vi "DFD FXP MRate Modeling.vi"(4 "internal precision":T3, 5 "output integer word length":T1, 6 "output rounding mode":T2=enum."Truncation", 7 "input integer word length":i16=1, 8 "error in (no error)":errorcluster, 9 "output word length":i16=16, 10 "input word length":i16=16, 11 "multirate filter in":T4={"mMRate_Structure"=enum."IIR", "mMRate_Mode"=0, "mMRate_Factor"=-1, "mMRate_FIRParams"={"mMRate_FIR_H"=[], "mMRate_FIR_IsNyquist?"=FALSE, "mMRate_FIR_IsSymmetric?"=FALSE}, "mMRate_CICParams"={"mMRate_CIC_#Stage"=0, "mMRate_CIC_Lag"=0, "mMRate_CIC_Type"=enum."Lowpass"}, "mMRate_Order"=0, "mMRate_Version"="2.0", "mMRate_Comments"="", "mMRate_RationalFactor"={"mMRate_L"=-1, "mMRate_M"=-1}, "mMRate_Fs"=1.0, "mMRate_Quantized?"=FALSE, "mMRate_QFilterGain"=1.0, "mMRate_CoefWl"=16, "mMRate_Scaling"={"mMRate_ScaleByPowerOf2?"=FALSE, "mMRate_ScaleType"=enum."No Norm"}, "mMRate_InputWl"=16, "mMRate_OutputWl"=16, "mMRate_OutputMode"=enum."Truncation", "mMRate_MultMode"=enum."Truncated", "mMRate_BitPruning"=FALSE, "mMRate_GainWl"=16, "mMRate_OutputFwl"=0, "mMRate_SumIwl"=0, "mMRate_InputIwl "=16, "mMRate_SumWl"=32, "mMRate_CoefIwl"=0} {"mMRate_SumWl" min=1 max=32 step=1; "mMRate_InputIwl" min=1 max=32 step=1; "mMRate_GainWl" min=1 max=32 step=1; "mMRate_OutputWl" min=1 max=32 step=1; "mMRate_InputWl" min=1 max=32 step=1; "mMRate_CoefWl" min=1 max=32 step=1; "mMRate_Mode" items=["Default"=-1, "No Rate Change"=0, "Interpolation"=1, "Decimation"=2, "Interpolated"=3, "Rational"=4]}) -> (0 "error out":errorcluster, 3 "multirate filter out":T4={"mMRate_Structure"=enum."IIR", "mMRate_Mode"=0, "mMRate_Factor"=-1, "mMRate_FIRParams"={"mMRate_FIR_H"=[], "mMRate_FIR_IsNyquist?"=FALSE, "mMRate_FIR_IsSymmetric?"=FALSE}, "mMRate_CICParams"={"mMRate_CIC_#Stage"=0, "mMRate_CIC_Lag"=0, "mMRate_CIC_Type"=enum."Lowpass"}, "mMRate_Order"=0, "mMRate_Version"="2.0", "mMRate_Comments"="", "mMRate_RationalFactor"={"mMRate_L"=-1, "mMRate_M"=-1}, "mMRate_Fs"=1.0, "mMRate_Quantized?"=FALSE, "mMRate_QFilterGain"=1.0, "mMRate_CoefWl"=16, "mMRate_Scaling"={"mMRate_ScaleByPowerOf2?"=FALSE, "mMRate_ScaleType"=enum."No Norm"}, "mMRate_InputWl"=16, "mMRate_OutputWl"=16, "mMRate_OutputMode"=enum."Truncation", "mMRate_MultMode"=enum."Truncated", "mMRate_BitPruning"=FALSE, "mMRate_GainWl"=16, "mMRate_OutputFwl"=0, "mMRate_SumIwl"=0, "mMRate_InputIwl "=16, "mMRate_SumWl"=32, "mMRate_CoefIwl"=0} {"mMRate_SumWl" min=1 max=32 step=1; "mMRate_InputIwl" min=1 max=32 step=1; "mMRate_GainWl" min=1 max=32 step=1; "mMRate_OutputWl" min=1 max=32 step=1; "mMRate_InputWl" min=1 max=32 step=1; "mMRate_CoefWl" min=1 max=32 step=1; "mMRate_Mode" items=["Default"=-1, "No Rate Change"=0, "Interpolation"=1, "Decimation"=2, "Interpolated"=3, "Rational"=4]})   [LabVIEW 2017, in "NI_DigFilterLicensed.lvlib"]
doc: "Creates a fixed-point multirate filter model according to the settings of the input word length, input integer word length, and output word length."
uses:
  <vilib>/addons/Digital Filter Design/NI_DigFilterLicensed.lvlib
  <vilib>/addons/Digital Filter Design/_Objects.llb/DFD Multirate Filter Obj.ctl
  <vilib>/addons/Digital Filter Design/_Objects.llb/DFD Multirate Mode.ctl
  <vilib>/addons/Digital Filter Design/_Objects.llb/DFD Coef Norm Type.ctl
  <vilib>/addons/Digital Filter Design/_Objects.llb/DFD Round-off Mode.ctl
  <vilib>/addons/Digital Filter Design/_Objects.llb/DFD FXP MRate Multiply Mode.ctl
  <vilib>/addons/Digital Filter Design/_Objects.llb/DFD FXP MRate Internal Precision Mode.ctl
  <vilib>/addons/Digital Filter Design/_Objects.llb/DFD Output Iwl Obj.ctl
  <vilib>/addons/Digital Filter Design/_Misc.llb/dfd_Error Handlers (Single).vi
  <vilib>/addons/Digital Filter Design/NI_DigFilter_FXP.lvlib
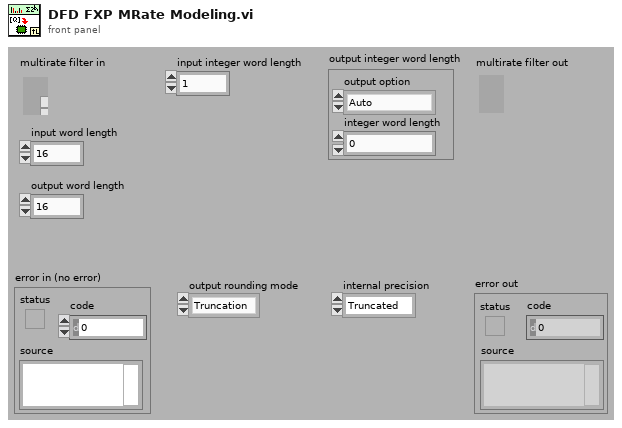
[diagram p1: front panel]
types:
  T1 = typedef "NI_DigFilterLicensed.lvlib/DFD Output Iwl Obj.ctl" = cluster{"output option":enum16{"Auto", "Same As Input", "User Defined"}, "integer word length":i16}
  T2 = typedef "NI_DigFilterLicensed.lvlib/DFD Round-off Mode.ctl" = enum16{"Nearest", "Truncation"}
  T3 = typedef "NI_DigFilterLicensed.lvlib/DFD FXP MRate Internal Precision Mode.ctl" = enum16{"Truncated", "Full"}
  T4 = typedef "NI_DigFilterLicensed.lvlib/DFD Multirate Filter Obj.ctl" = cluster{"mMRate_Structure":enum16{"CIC", "FIR", "IIR", "Lattice"}, "mMRate_Mode":T5, "mMRate_Factor":i32, "mMRate_FIRParams":cluster{"mMRate_FIR_H":dbl[], "mMRate_FIR_IsNyquist?":bool, "mMRate_FIR_IsSymmetric?":bool}, "mMRate_CICParams":cluster{"mMRate_CIC_#Stage":i32, "mMRate_CIC_Lag":i32, "mMRate_CIC_Type":enum16{"Lowpass", "Highpass"}}, "mMRate_Order":i32, "mMRate_Version":string, "mMRate_Comments":string, "mMRate_RationalFactor":cluster{"mMRate_L":i32, "mMRate_M":i32}, "mMRate_Fs":dbl, "mMRate_Quantized?":bool, "mMRate_QFilterGain":dbl, "mMRate_CoefWl":i16, "mMRate_Scaling":cluster{"mMRate_ScaleByPowerOf2?":bool, "mMRate_ScaleType":T6}, "mMRate_InputWl":i16, "mMRate_OutputWl":i16, "mMRate_OutputMode":T2, "mMRate_MultMode":T7, "mMRate_BitPruning":bool, "mMRate_GainWl":i16, "mMRate_OutputFwl":i16, "mMRate_SumIwl":i16, "mMRate_InputIwl ":i16, "mMRate_SumWl":i16, "mMRate_CoefIwl":i16}
  T5 = typedef "NI_DigFilterLicensed.lvlib/DFD Multirate Mode.ctl" = i16
  T6 = typedef "NI_DigFilterLicensed.lvlib/DFD Coef Norm Type.ctl" = enum16{"No Norm", "Time Domain 1-Norm", "Time Domain 2-Norm", "Time Domain Inf-Norm"}
  T7 = typedef "NI_DigFilterLicensed.lvlib/DFD FXP MRate Multiply Mode.ctl" = enum16{"Truncated", "Full"}
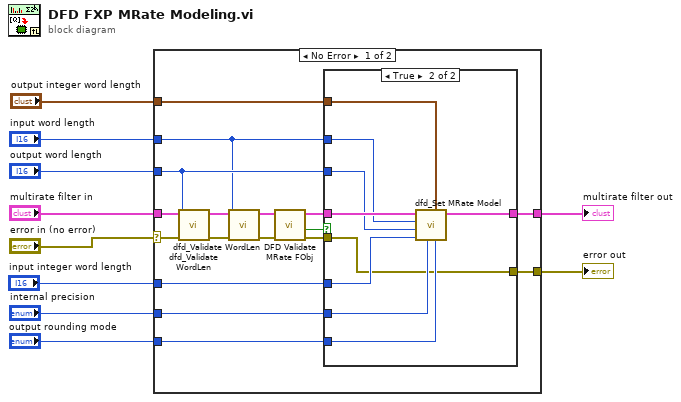
[diagram p0: block diagram]
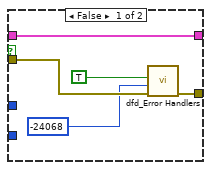
[diagram p2: hidden frame]
diagram:
  n1 = case shown="No Error" "error in (no error)" {
    selector: "error in (no error)" -> [w12 w40]
    tunnel: [w23 _] -> w10
    tunnel: [w22 w40] -> w9
    tunnel: "output word length" -> [w20 _]
    tunnel: "input word length" -> [w19 _]
    tunnel: "internal precision" -> [w17 _]
    tunnel: "output rounding mode" -> [w16 _]
    tunnel: "multirate filter in" -> [w15 _]
    tunnel: "input integer word length" -> [w13 _]
    tunnel: "output integer word length" -> [w11 _]
    frame No Error {
      n2 = call <vilib>:"dfd_Validate WordLen.vi"("error in (no error)"=w12, "wl"=w20) -> ("error out"=w21:errorcluster)  [unwired: 9 out]
      n3 = call <vilib>:"dfd_Validate WordLen.vi"("error in (no error)"=w21, "wl"=w19) -> ("error out"=w14:errorcluster)  [unwired: 9 out]
      n4 = call <vilib>:"DFD Validate MRate FObj.vi"("error in (no error)"=w14, "multirate filter in"=w15) -> ("error out"=w24:errorcluster, "is valid FXP?"=w18:bool, "multirate filter out"=w25:T4)  [unwired: 7 out]
      n5 = case shown="True" w18 {
        tunnel: w25 -> [w26 w39]
        tunnel: w24 -> [w29 w32]
        tunnel: w19 -> [_ w37]
        tunnel: w20 -> [_ w38]
        tunnel: [w26 w34] -> w23
        tunnel: [w30 w32] -> w22
        tunnel: w17 -> [_ w36]
        tunnel: w16 -> [_ w35]
        tunnel: w13 -> [_ w33]
        tunnel: w11 -> [_ w31]
        frame False {
          n6 = call-poly <vilib>:"dfd_Error Handlers.vi"("error in (no error)"=w29, "error code"=-24068 ("ERR_INVALID_FXP_MRATE"), "condition failed?"=TRUE) -> ("error out"=w30:errorcluster)  [unwired: 8 out]
        }
        frame True {
          n7 = call <vilib>:"dfd_Set MRate Model.vi"("output rounding mode"=w35, "output integer word length"=w31, "internal precision"=w36, "input iwl"=w33, "output wl"=w38, "input wl"=w37, "multirate filter in"=w39) -> ("multirate filter out"=w34:T4)  [unwired: 4 out]
        }
      }
    }
    frame Error {
    }
  }
  "multirate filter out" <- w10
  "error out" <- w9
